vi "10 DAQ Config (PFI0) (x64-2018).vi"(2 "Error In":errorcluster, 3 "rate":dbl=6000.0, 4 "number of samples":i32=240) -> (0 "Error Out":errorcluster, 1 "task out":refnum<k21>)   [LabVIEW 2017]
uses:
  <vilib>/DAQmx/create/channels.llb/DAQmx Create Channel (TEDS-AI-Voltage-Basic).vi
  <vilib>/DAQmx/create/channels.llb/DAQmx Create Channel (AI-Voltage-Basic).vi
  <vilib>/DAQmx/configure/timing.llb/DAQmx Timing (Sample Clock).vi
  <vilib>/DAQmx/configure/trigger.llb/DAQmx Trigger.vi
  <vilib>/DAQmx/configure/trigger.llb/DAQmx Start Trigger (Digital Edge).vi
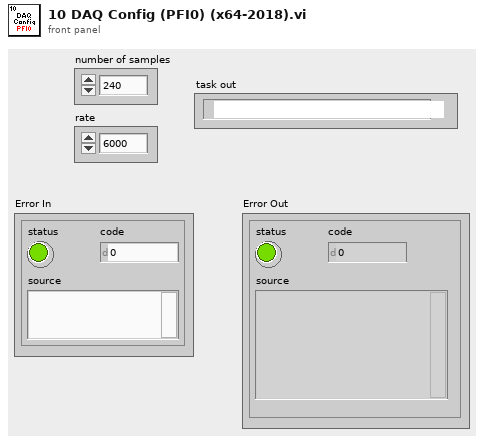
[diagram p1: front panel]
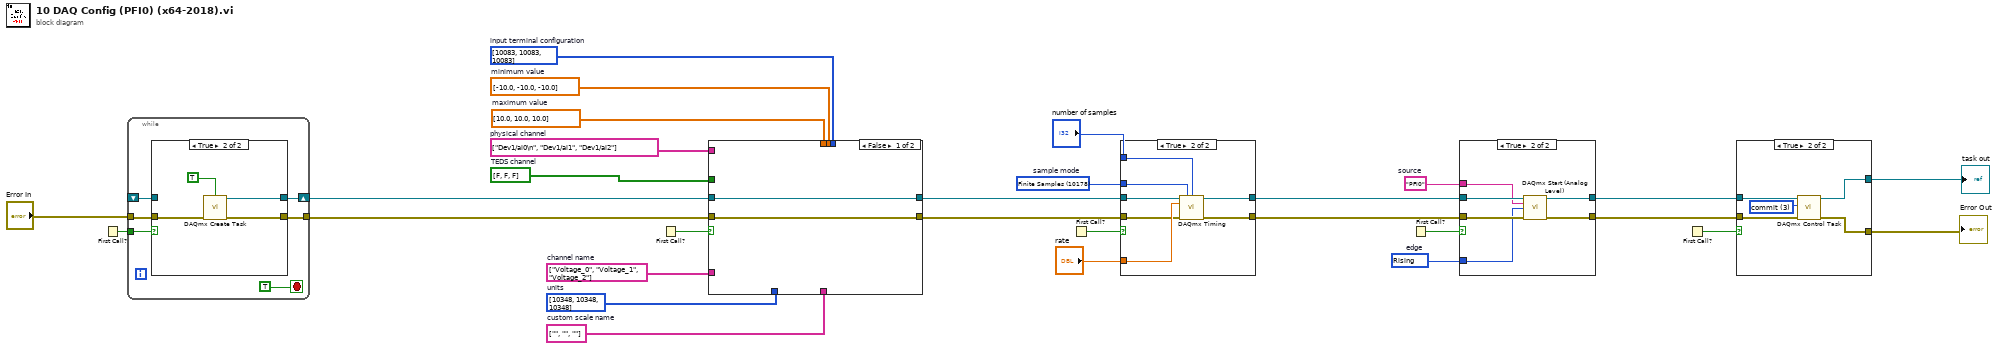
[diagram p0: block diagram]
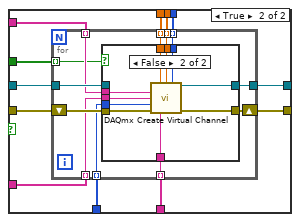
[diagram p5: hidden frame]
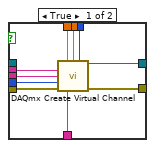
[diagram p6: hidden frame]
diagram:
  w26 = 10280 items=["Rising"=10280, "Falling"=10171]  # edge
  w25 = "PFI0"  # source
  w21 = 10178 items=["Finite Samples"=10178, "Continuous Samples"=10123, "Hardware Timed Single Point"=12522]  # sample mode
  w15 = bool[] [FALSE, FALSE, FALSE]  # TEDS channel
  w14 = string[] ["", "", ""]  # custom scale name
  w13 = i32[] [10348, 10348, 10348] items=["Volts"=10348, "From TEDS"=12516, "From Custom Scale"=10065]  # units
  w12 = string[] ["Voltage_0", "Voltage_1", "Voltage_2"]  # channel name
  w11 = string[] ["Dev1/ai0\n", "Dev1/ai1", "Dev1/ai2"]  # physical channel
  w10 = dbl[] [10.0, 10.0, 10.0]  # maximum value
  w9 = dbl[] [-10.0, -10.0, -10.0]  # minimum value
  w8 = i32[] [10083, 10083, 10083] items=["default"=-1, "RSE"=10083, "NRSE"=10078, "Differential"=10106, "Pseudodifferential"=12529]  # input terminal configuration
  n1 = First Call?() -> (First Call?: T/F=w3:bool)
  n2 = while {
    shift-right: [w34] -> w6
    shift-left: _ -> [w33]
    tunnel: w3 -> [w35]
    tunnel: [w32] -> w4
    tunnel: "Error In" -> [w31]
    stop <- TRUE stop-if-true
    n3 = case shown="True" w35 {
      tunnel: [w37 w38] -> w34
      tunnel: w33 -> [w37 _]
      tunnel: [w36 w41] -> w32
      tunnel: w31 -> [w36 w39]
      frame False {
      }
      frame True {
        n4 = call <vilib>:"DAQmx Create Task.vi"("auto cleanup"=TRUE, "error in"=w39) -> ("task out"=w38:refnum<k21>, "error out"=w41:errorcluster)  [unwired: 12 in]
      }
    }
  }
  n5 = First Call?() -> (First Call?: T/F=w5:bool)
  n6 = case shown="False" w5 {
    tunnel: [w42 w53] -> w17
    tunnel: w6 -> [w42 w55]
    tunnel: [w43 w52] -> w7
    tunnel: w4 -> [w43 w54]
    tunnel: w8 -> [_ w51]
    tunnel: w9 -> [_ w50]
    tunnel: w10 -> [_ w49]
    tunnel: w11 -> [_ w48]
    tunnel: w12 -> [_ w47]
    tunnel: w13 -> [_ w46]
    tunnel: w14 -> [_ w45]
    tunnel: w15 -> [_ w44]
    frame False {
    }
    frame True {
      n7 = for {
        tunnel: w55 -> [w67]
        tunnel: [w65] -> w53
        tunnel: w51 -> [w63] mode=indexing
        tunnel: w50 -> [w62] mode=indexing
        tunnel: w49 -> [w61] mode=indexing
        tunnel: w48 -> [w60] mode=indexing
        tunnel: w47 -> [w59] mode=indexing
        tunnel: w46 -> [w58] mode=indexing
        tunnel: w45 -> [w57] mode=indexing
        shift-right: [w64] -> w52
        shift-left: w54 -> [w66]
        tunnel: w44 -> [w56] mode=indexing
        n8 = case shown="False" w56 {
          tunnel: w67 -> [_ _]
          tunnel: w66 -> [w77 w87]
          tunnel: [w76 w86] -> w65
          tunnel: [w75 w85] -> w64
          tunnel: w63 -> [w74 w84]
          tunnel: w62 -> [w73 w83]
          tunnel: w61 -> [w72 w82]
          tunnel: w60 -> [w71 w81]
          tunnel: w59 -> [w70 w80]
          tunnel: w58 -> [w69 w79]
          tunnel: w57 -> [w68 w78]
          frame True {
            n9 = call-poly <vilib>:"DAQmx Create Virtual Channel.vi"("maximum value"=w72, "minimum value"=w73, "input terminal configuration"=w74, "physical channels"=w71, "name to assign"=w70, "units"=w69, "error in"=w77, "custom scale name"=w68) -> ("task out"=w76:refnum<k21>, "error out"=w75:errorcluster)  [unwired: 6 in]
          }
          frame False {
            n10 = call-poly <vilib>:"DAQmx Create Virtual Channel.vi"("maximum value"=w82, "minimum value"=w83, "input terminal configuration"=w84, "physical channels"=w81, "name to assign"=w80, "units"=w79, "error in"=w87, "custom scale name"=w78) -> ("task out"=w86:refnum<k21>, "error out"=w85:errorcluster)  [unwired: 6 in]
          }
        }
      }
    }
  }
  n11 = First Call?() -> (First Call?: T/F=w16:bool)
  n12 = case shown="True" w16 {
    tunnel: [w89 w91] -> w23
    tunnel: w17 -> [w89 w94]
    tunnel: [w88 w90] -> w18
    tunnel: w7 -> [w88 w92]
    tunnel: "number of samples" -> [_ w96]
    tunnel: w21 -> [_ w95]
    tunnel: "rate" -> [_ w93]
    frame False {
    }
    frame True {
      n13 = call-poly <vilib>:"DAQmx Timing.vi"("task/channels in"=w94, "sample mode"=w95, "samples per channel"=w96, "rate"=w93, "error in"=w92) -> ("task out"=w91:refnum<k21>, "error out"=w90:errorcluster)  [unwired: 9 in]
    }
  }
  n14 = First Call?() -> (First Call?: T/F=w22:bool)
  n15 = case shown="True" w22 {
    tunnel: [w98 w102] -> w28
    tunnel: w23 -> [w98 w104]
    tunnel: [w97 w101] -> w24
    tunnel: w18 -> [w97 w103]
    tunnel: w25 -> [_ w100]
    tunnel: w26 -> [_ w99]
    frame False {
    }
    frame True {
      n16 = call-poly "DAQmx Start (Analog Level).vi"("task/channels in"=w104, "source"=w100, "edge"=w99, "error in"=w103) -> ("task out"=w102:refnum<k21>, "error out"=w101:errorcluster)  [unwired: 10 in]
    }
  }
  n17 = First Call?() -> (First Call?: T/F=w27:bool)
  n18 = case shown="True" w27 {
    tunnel: [w106 w110] -> w29
    tunnel: w28 -> [w106 w111]
    tunnel: [w105 w108] -> w1
    tunnel: w24 -> [w105 w109]
    frame False {
    }
    frame True {
      w107 = 3 items=["verify"=2, "reserve"=4, "commit"=3, "unreserve"=5, "abort"=6] ("action")
      n19 = call <vilib>:"DAQmx Control Task.vi"("task/channels in"=w111, "action"=w107, "error in"=w109) -> ("task out"=w110:refnum<k21>, "error out"=w108:errorcluster)  [unwired: 11 in]
    }
  }
  "task out" <- w29
  "Error Out" <- w1
